vi "WRITE.vi"(1 "Data to Write":u8[](array[numeric])=[0, 0, 0, 0, 0, 0, 0, 0] format="%02x", 2 "Frames to Write":u8, 3 "Starting Address":u8 format="%02x", 4 "SPI Config In":T1) -> (0 "SPI Config Out":T1)   [LabVIEW 2019]
uses:
  SPI/SPI Config.ctl
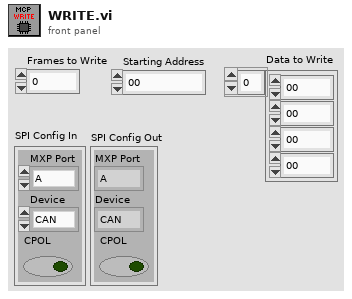
[diagram p1: front panel]
types:
  T1 = typedef "SPI Config.ctl" = cluster{"MXP Port":enum16{"A", "B"}, "Device":enum16{"CAN", "ENC", "IMU1", "IMU2"}, "CPOL":bool}
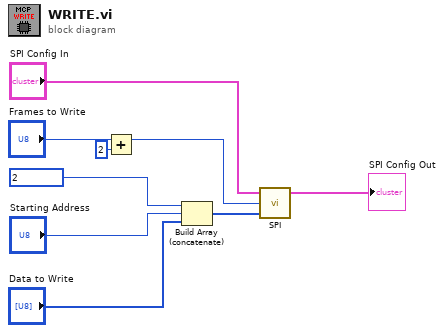
[diagram p0: block diagram]
diagram:
  n1 = Add(x="Frames to Write", y=u8 2) -> (x+y=w4:u8)
  n2 = Build Array (concatenate)(u8 2, "Starting Address", "Data to Write") -> (w6:u8[])
  n3 = call "SPI.vi"("Data to Write"=w6, "Frames to Write"=w4, "SPI Config In"="SPI Config In") -> ("SPI Config Out"=→"SPI Config Out":T1)  [unwired: 2 out]
